vi "Measure Voltage.vi"(8 "error in (no error)":errorcluster, 11 "DMM_Concrete in":refnum<class "DMM_Concrete.lvclass">) -> (0 "error out":errorcluster, 2 "Voltage (V)":dbl, 3 "DMM_Concrete out":refnum<class "DMM_Concrete.lvclass">)   [LabVIEW 2024, in "HAL_Example.lvlib" / "DMM_Concrete.lvclass"]
uses:
  DMM/DMM_Concrete.lvclass
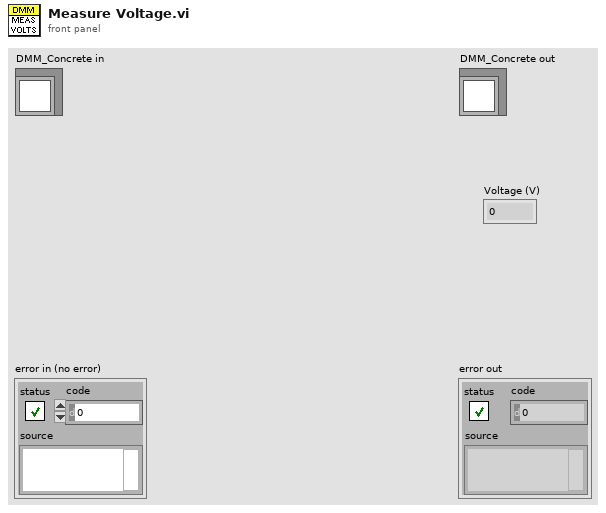
[diagram p1: front panel]
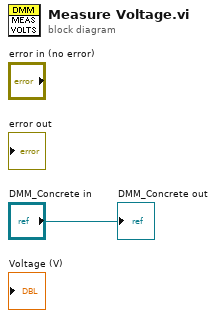
[diagram p0: block diagram]
diagram:
  "DMM_Concrete out" <- "DMM_Concrete in"
